vi "Post Process Noise Filter.vi"(0 "pInputImage":i32, 1 "iMode":i32, 2 "iHeight":i32, 5 "pOutputImage":i32, 7 "iOutputBufferSize":i32, 9 "iBaseline":i32, 12 "fThreshold":sgl, 13 "iWidth":i32) -> (4 "pInputImage out":i32, 6 "pOutputImage out":i32, 8 "function return":u32)   [LabVIEW 2018, in "Copy of Andor SDK.lvlib"]
doc: "EXPNETTYPE unsigned int WINAPI PostProcessNoiseFilter(at_32 * pInputImage, at_32 * pOutputImage, int iOutputBufferSize, int iBaseline, int iMode, float fThreshold, int iHeight, int iWidth);"
uses:
  Copy of Andor SDK.lvlib
  <userlib>/Andor SDK/ATMCD32D.dll
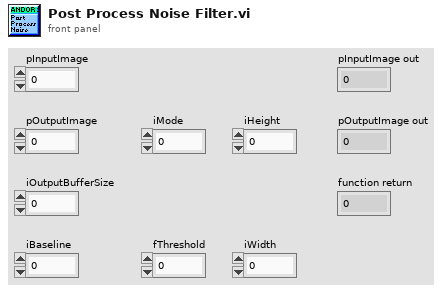
[diagram p1: front panel]
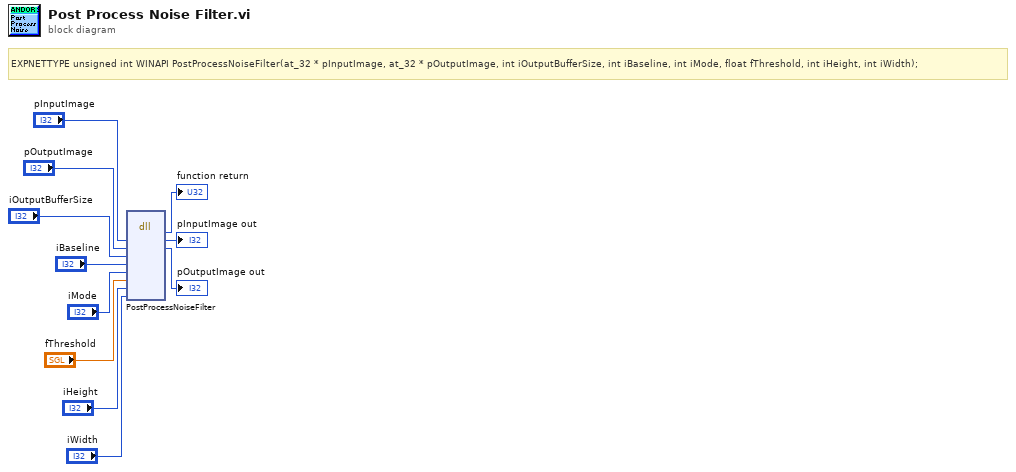
[diagram p0: block diagram]
diagram:
  # "EXPNETTYPE unsigned int WINAPI PostProcessNoiseFilter(at_32 * pInputImage, at_32 * pOutputImage, int iOutputBufferSize, int iBaseline, int iMode, float fThreshold, int iHeight, int iWidth);"
  n1 = dll-call lib="C:/Program Files (x86)/National Instruments/LabVIEW 2018/user.lib/Andor SDK/ATMCD32D.*" fn="PostProcessNoiseFilter"("pInputImage"="pInputImage", "pOutputImage"="pOutputImage", "iOutputBufferSize"="iOutputBufferSize", "iBaseline"="iBaseline", "iMode"="iMode", "fThreshold"="fThreshold", "iHeight"="iHeight", "iWidth"="iWidth") -> (→"function return":u32, "pInputImage"=→"pInputImage out":i32, "pOutputImage"=→"pOutputImage out":i32)  [unwired: 9 in, 2 out]
